vi "SQLite Delete Saving Test.vi"(7 "Test DB Set Up Command":string, 8 "Error In (no error)":errorcluster, 11 "SQLite DB Operator In":refnum<class "SQLite DB Operator.lvclass">) -> (0 "Error Out":errorcluster, 3 "SQLite DB Operator Out":refnum<class "SQLite DB Operator.lvclass">)   [LabVIEW 2023]
uses:
  Clasess/SQLite DB Operator/SQLite DB Operator.lvclass
  Clasess/DB Records/Expenses Tracker Saving/Public/Ctrls/Saving.ctl
  Clasess/DB Records/Expenses Tracker Saving/Expenses Tracker Saving.lvclass
  H:/Desktop/LabVIEW/LabView Repo/Expenses-Tracker-DB-Operator/Interfaces/Expenses Tracker Record/Expenses Tracker Record.lvclass
  Support/Editing/Edit Record Assert Error.vi
  Support/Editing/Edit Record Assert Not Error.vi
  <vilib>/drjdpowell/SQLite Library/SQL Connection/Execute SQL (1D Cluster).vi
  <vilib>/addons/_JKI Toolkits/Caraya/classes/Test/Test.lvclass
  <vilib>/drjdpowell/SQLite Library/SQLite.lvlib
  H:/Desktop/LabVIEW/LabView Repo/Expenses-Tracker-DB-Operator/Clasess/DB Records/Expenses Tracker Saving/Expenses Tracker Saving.lvclass
  <vilib>/drjdpowell/SQLite Library/SQL Connection/Connection.lvclass
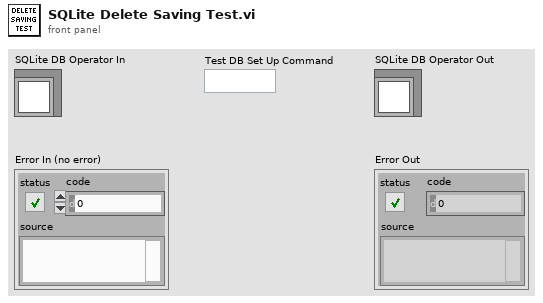
[diagram p1: front panel]
types:
  T1 = typedef "Expenses Tracker Saving.lvclass/Saving.ctl" = cluster{"ID":u32, "Saving_goal":u32, "Value":dbl, "Date_of_entry":timestamp, "Description":string}
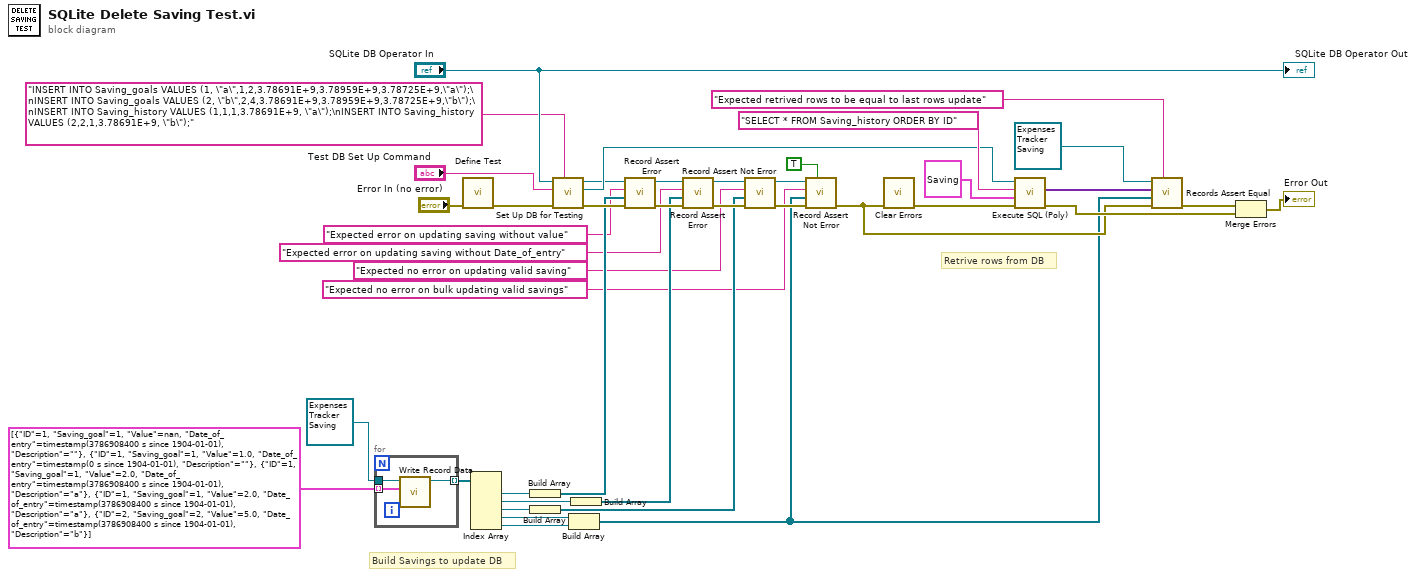
[diagram p0: block diagram]
diagram:
  # "Retrive rows from DB"
  # "Build Savings to update DB"
  n1 = for {
    tunnel: T1[] [{"ID"=1, "Saving_goal"=1, "Value"=nan, "Date_of_entry"=timestamp(3786908400 s since 1904-01-01), "Description"=""}, {"ID"=1, "Saving_goal"=1, "Value"=1.0, "Date_of_entry"=timestamp(0 s since 1904-01-01), "Description"=""}, {"ID"=1, "Saving_goal"=1, "Value"=2.0, "Date_of_entry"=timestamp(3786908400 s since 1904-01-01), "Description"="a"}, {"ID"=1, "Saving_goal"=1, "Value"=2.0, "Date_of_entry"=timestamp(3786908400 s since 1904-01-01), "Description"="a"}, {"ID"=2, "Saving_goal"=2, "Value"=5.0, "Date_of_entry"=timestamp(3786908400 s since 1904-01-01), "Description"="b"}] ("Array") -> [w44] mode=indexing
    tunnel: refnum<class "Expenses Tracker Saving.lvclass"> refnum ("Expenses Tracker Category") -> [w42]
    tunnel: [w43] -> w39 mode=indexing
    n2 = call-dynamic "Write Record Data.vi"("Record"=w44, "Expenses Tracker Saving In"=w42) -> ("Expenses Tracker Saving Out"=w43:refnum<class "Expenses Tracker Saving.lvclass">)  [unwired: 8 in, 1 out]
  }
  n3 = call <vilib>:"Define Test.vi"("error in (no error)"="Error In (no error)") -> ("error out"=w33:errorcluster)  [unwired: 9 in, 1 out]
  n4 = Index Array(array=w39) -> (element #1=w22:refnum<class "Expenses Tracker Saving.lvclass">, element #2=w18:refnum<class "Expenses Tracker Saving.lvclass">, element #3=w15:refnum<class "Expenses Tracker Saving.lvclass">, element #4=w5:refnum<class "Expenses Tracker Saving.lvclass">, element #5=w4:refnum<class "Expenses Tracker Saving.lvclass">)  [unwired: 5 in]
  n5 = Build Array(w22) -> (w21:refnum<class "Expenses Tracker Saving.lvclass">[])
  n6 = Build Array(w15) -> (w10:refnum<class "Expenses Tracker Saving.lvclass">[])
  n7 = call "Set Up DB for Testing.vi"("Additional Set Up Commands"="INSERT INTO Saving_goals VALUES (1, \"a\",1,2,3.78691E+9,3.78959E+9,3.78725E+9,\"a\");\nINSERT INTO Saving_goals VALUES (2, \"b\",2,4,3.78691E+9,3.78959E+9,3.78725E+9,\"b\");\nINSERT INTO Saving_history VALUES (1,1,1,3.78691E+9, \"a\");\nINSERT INTO Saving_history VALUES (2,2,1,3.78691E+9, \"b\");", "Error In (no error)"=w33, "Test DB Set Up Command"="Test DB Set Up Command", "SQLite DB Operator In"="SQLite DB Operator In") -> ("Error Out"=w23:errorcluster, "SQLite Connection"=w36:refnum<class "Connection.lvclass">, "SQLite DB Operator Out"=w20:refnum<class "SQLite DB Operator.lvclass">)  [unwired: 5 in]
  n8 = Build Array(w5, w4) -> (w2:refnum<class "Expenses Tracker Saving.lvclass">[])
  n9 = Build Array(w18) -> (w17:refnum<class "Expenses Tracker Saving.lvclass">[])
  n10 = call-poly "Record Assert Error.vi"("Error In"=w23, "Records"=w21, "Assertion Label"="Expected error on updating saving without value" ("Label (VI Title)"), "SQLite DB Operator In"=w20) -> ("Error Out"=w26:errorcluster, "SQLite DB Operator Out"=w27:refnum<class "SQLite DB Operator.lvclass">)  [unwired: 6 in]
  n11 = call-poly "Record Assert Error.vi"("Error In"=w26, "Records"=w17, "Assertion Label"="Expected error on updating saving without Date_of_entry" ("Label (VI Title)"), "SQLite DB Operator In"=w27) -> ("Error Out"=w24:errorcluster, "SQLite DB Operator Out"=w25:refnum<class "SQLite DB Operator.lvclass">)  [unwired: 6 in]
  n12 = call-poly "Record Assert Not Error.vi"("Error In"=w24, "Records"=w10, "Assertion Label"="Expected no error on updating valid saving" ("Label (VI Title)"), "SQLite DB Operator In"=w25) -> ("Error Out"=w8:errorcluster, "SQLite DB Operator Out"=w3:refnum<class "SQLite DB Operator.lvclass">)  [unwired: 6 in]
  n13 = call-poly "Record Assert Not Error.vi"("Bulk Update?"=TRUE, "Error In"=w8, "Records"=w2, "Assertion Label"="Expected no error on bulk updating valid savings" ("Label (VI Title)"), "SQLite DB Operator In"=w3) -> ("Error Out"=w6:errorcluster)  [unwired: 5 in, 1 out]
  n14 = call <vilib>:"Clear Errors.vi"("error in (no error)"=w6) -> ("error out"=w28:errorcluster)  [unwired: 5 in, 1 out]
  n15 = call-poly <vilib>:"Execute SQL (Poly).vi"("error in (no error)"=w28, "Cluster (or Array of Clusters)"=T1 {"ID"=0, "Saving_goal"=0, "Value"=0.0, "Date_of_entry"=timestamp(0 s since 1904-01-01), "Description"=""} ("Saving"), "SQL"="SELECT * FROM Saving_history ORDER BY ID", "SQLite Connection in"=w36) -> ("error out"=w29:errorcluster, "Result Set (Array of Clusters)"=w14:variant[])  [unwired: 5 in, 1 out]
  n16 = call "Records Assert Equal.vi"("Assertion Label"="Expected retrived rows to be equal to last rows update" ("Label (VI Title)"), "Error In"=w6, "Correct Records"=w2, "Typedef Records"=w14, "Expenses Tracker Record In"=refnum<class "Expenses Tracker Saving.lvclass"> refnum ("Expenses Tracker Category")) -> ("Error Out"=w30:errorcluster)  [unwired: 6 in]
  n17 = Merge Errors(w30, w29) -> (→"Error Out":errorcluster)
  "SQLite DB Operator Out" <- "SQLite DB Operator In"
